vi "Panel.IsOpen.vi"(1 "FP State":T1(ring)) -> (0 "Open?":bool)   [LabVIEW 2016]
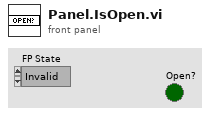
[diagram p1: front panel]
types:
  T1 = enum32{"Invalid", "Standard", "Closed", "Hidden", "Minimized", "Maximized"}
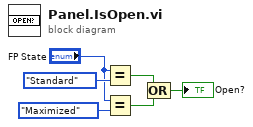
[diagram p0: block diagram]
diagram:
  n1 = Equal?(x="FP State", y=T1."Standard") -> (x = y?=w3:bool)
  n2 = Equal?(x="FP State", y=T1."Maximized") -> (x = y?=w2:bool)
  n3 = Compound Arithmetic op=OR(w3, w2) -> (→"Open?":bool)
